vi "gm_mysql_write_gmvalues.vi"(7 "db connection":bool, 8 "error in (no error)":errorcluster, 10 "Output - Cluster gm":T3 {"GM TS-2[°C]" format="%.2g"; "GM TS-1 [°C]" format="%.2g"; "GM DS-1 [bar]" format="%.4g"; "GM DS-2 [bar]" format="%.4g"; "GA1 h2 [%]" format="%.2g"; "GA1 co2 [%]" format="%.2g"; "GA1 ch4 [%]" format="%.2g"}, 11 "log vars in":T1) -> (0 "error out":errorcluster, 2 "db connection":bool, 3 "log vars out":T1)   [LabVIEW 2011]
uses:
  Output - Cluster gas.ctl
  gas_values.ctl
  GM_host_db_log_vars.ctl
  <vilib>/addons/database/Connection.llb/Conn ObjectReference.ctl
  <vilib>/Utility/error.llb/DialogType.ctl
  <vilib>/addons/database/NI_Database_API.lvlib
panel:
  # "qualitätsmessung"
  # "quantitätsmessung"
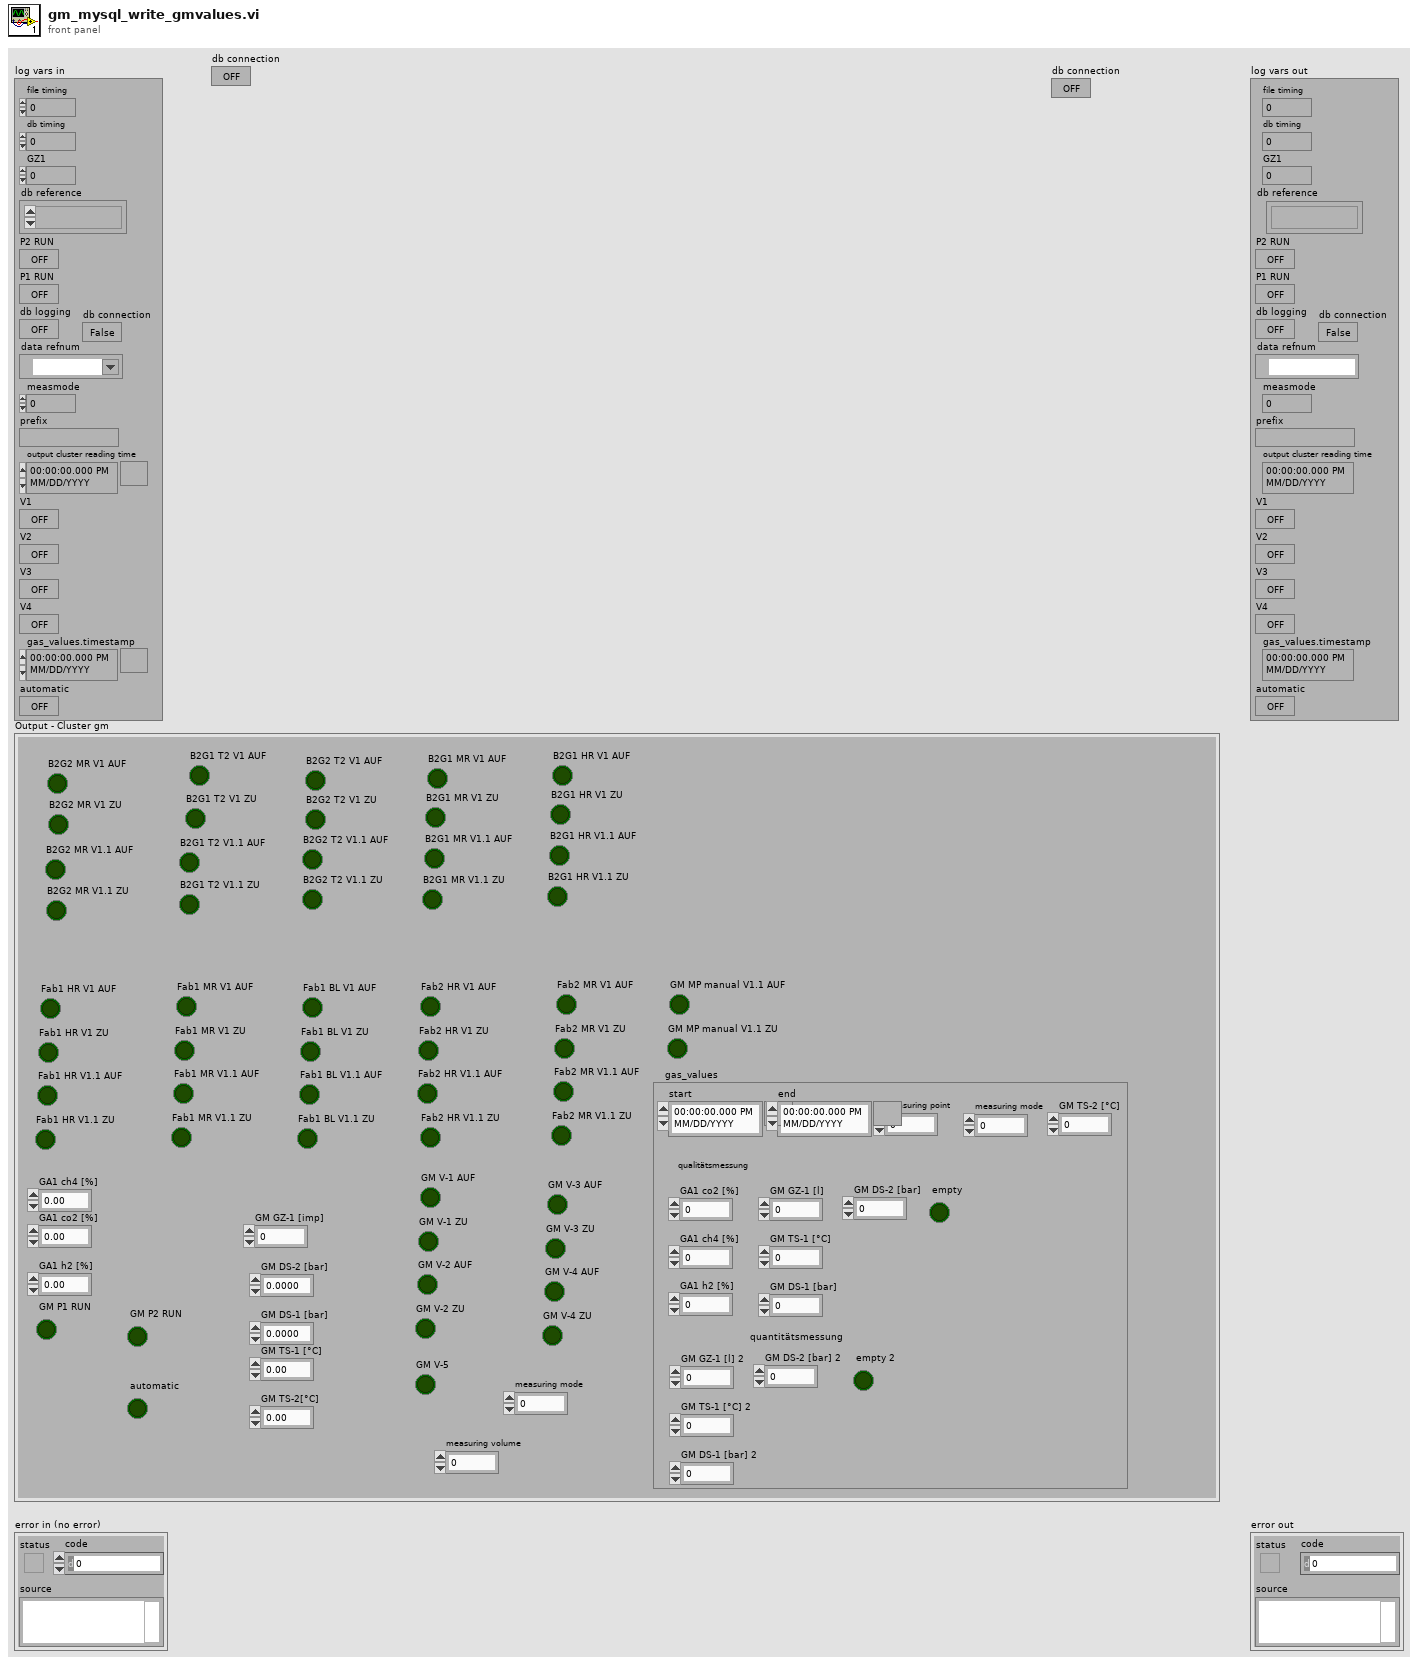
[diagram p1: front panel]
types:
  T1 = typedef "GM_host_db_log_vars.ctl" = cluster{"file timing":i64, "db timing":i64, "GZ1":u32, "db reference":T2, "P2 RUN":bool, "P1 RUN":bool, "db logging":bool, "data refnum":refnum<k21>, "measmode":u32, "prefix":string, "output cluster reading time":timestamp, "V1":bool, "V2":bool, "V3":bool, "V4":bool, "gas_values.timestamp":timestamp, "automatic":bool, "db connection":bool}
  T2 = typedef "NI_Database_API.lvlib/Conn ObjectReference.ctl" = refnum<k1>
  T3 = typedef "Output - Cluster gas.ctl" = cluster{"B2G2 MR V1.1 AUF":bool, "B2G2 MR V1.1 ZU":bool, "B2G2 MR V1 AUF":bool, "B2G2 MR V1 ZU":bool, "B2G1 T2 V1 AUF":bool, "B2G1 T2 V1 ZU":bool, "B2G1 T2 V1.1 AUF":bool, "B2G1 T2 V1.1 ZU":bool, "B2G2 T2 V1 AUF":bool, "B2G2 T2 V1 ZU":bool, "B2G2 T2 V1.1 ZU":bool, "B2G2 T2 V1.1 AUF":bool, "B2G1 MR V1 AUF":bool, "B2G1 MR V1 ZU":bool, "B2G1 MR V1.1 AUF":bool, "B2G1 MR V1.1 ZU":bool, "B2G1 HR V1 AUF":bool, "B2G1 HR V1 ZU":bool, "B2G1 HR V1.1 AUF":bool, "B2G1 HR V1.1 ZU":bool, "Fab1 HR V1 AUF":bool, "Fab1 HR V1 ZU":bool, "Fab1 HR V1.1 AUF":bool, "Fab1 HR V1.1 ZU":bool, "Fab1 MR V1 AUF":bool, "Fab1 MR V1 ZU":bool, "Fab1 MR V1.1 AUF":bool, "Fab1 MR V1.1 ZU":bool, "Fab1 BL V1 AUF":bool, "Fab1 BL V1 ZU":bool, "Fab1 BL V1.1 AUF":bool, "Fab1 BL V1.1 ZU":bool, "Fab2 HR V1 AUF":bool, "Fab2 HR V1 ZU":bool, "Fab2 HR V1.1 AUF":bool, "Fab2 HR V1.1 ZU":bool, "Fab2 MR V1 AUF":bool, "Fab2 MR V1 ZU":bool, "Fab2 MR V1.1 AUF":bool, "Fab2 MR V1.1 ZU":bool, "GA1 ch4 [%]":dbl, "GA1 co2 [%]":dbl, "GA1 h2 [%]":dbl, "GM P1 RUN":bool, "GM V-1 AUF":bool, "GM V-1 ZU":bool, "GM V-2 AUF":bool, "GM V-2 ZU":bool, "GM V-3 AUF":bool, "GM V-3 ZU":bool, "GM V-4 AUF":bool, "GM V-4 ZU":bool, "GM P2 RUN":bool, "GM GZ-1 [imp]":u32, "GM DS-2 [bar]":dbl, "GM DS-1 [bar]":dbl, "GM TS-1 [°C]":dbl, "GM TS-2[°C]":dbl, "gas_values":T4, "measuring mode":u8, "GM V-5":bool, "measuring volume":dbl, "automatic":bool, "GM MP manual V1.1 AUF":bool, "GM MP manual V1.1 ZU":bool}
  T4 = typedef "gas_values.ctl" = cluster{"start":timestamp, "GM DS-2 [bar]":dbl, "GA1 ch4 [%]":dbl, "GA1 co2 [%]":dbl, "GA1 h2 [%]":dbl, "GM DS-1 [bar]":dbl, "GM TS-1 [°C]":dbl, "GM TS-2 [°C]":dbl, "GM GZ-1 [l]":dbl, "measuring point":u8, "end":timestamp, "empty":bool, "GM GZ-1 [l] 2":dbl, "GM TS-1 [°C] 2":dbl, "GM DS-1 [bar] 2":dbl, "GM DS-2 [bar] 2":dbl, "empty 2":bool, "measuring mode":u8}
  T5 = typedef "DialogType.ctl" = u16
  T6 = cluster{"start":timestamp, "end":timestamp, "measuring point":u8, "measuring mode":u8, "GA1 co2 [%]":dbl, "GA1 ch4 [%]":dbl, "GA1 h2 [%]":dbl, "GM GZ-1 [l]":dbl, "GM DS-1 [bar]":dbl, "GM TS-1 [°C]":dbl, "GM DS-2 [bar]":dbl, i16, "GM TS-2 [°C]":dbl}
  T7 = cluster{"start":timestamp, "end":timestamp, "measuring point":u8, "measuring mode":u8, "GM GZ-1 [l] 2":dbl, "GM DS-1 [bar] 2":dbl, "GM TS-1 [°C] 2":dbl, "GM DS-2 [bar] 2":dbl, i16, "GM TS-2 [°C]":dbl}
  T8 = cluster{"start":timestamp, "end":timestamp, "measuring point":u8, "measuring mode":u8, "GA1 co2 [%]":dbl, "GA1 ch4 [%]":dbl, "GA1 h2 [%]":dbl, "GM GZ-1 [l]":dbl, "GM DS-1 [bar]":dbl, "GM TS-1 [°C]":dbl, "GM DS-2 [bar]":dbl, i16, "GM GZ-1 [l] 2":dbl, "GM DS-1 [bar] 2":dbl, "GM TS-1 [°C] 2":dbl, "GM DS-2 [bar] 2":dbl, i16, "GM TS-2 [°C]":dbl}
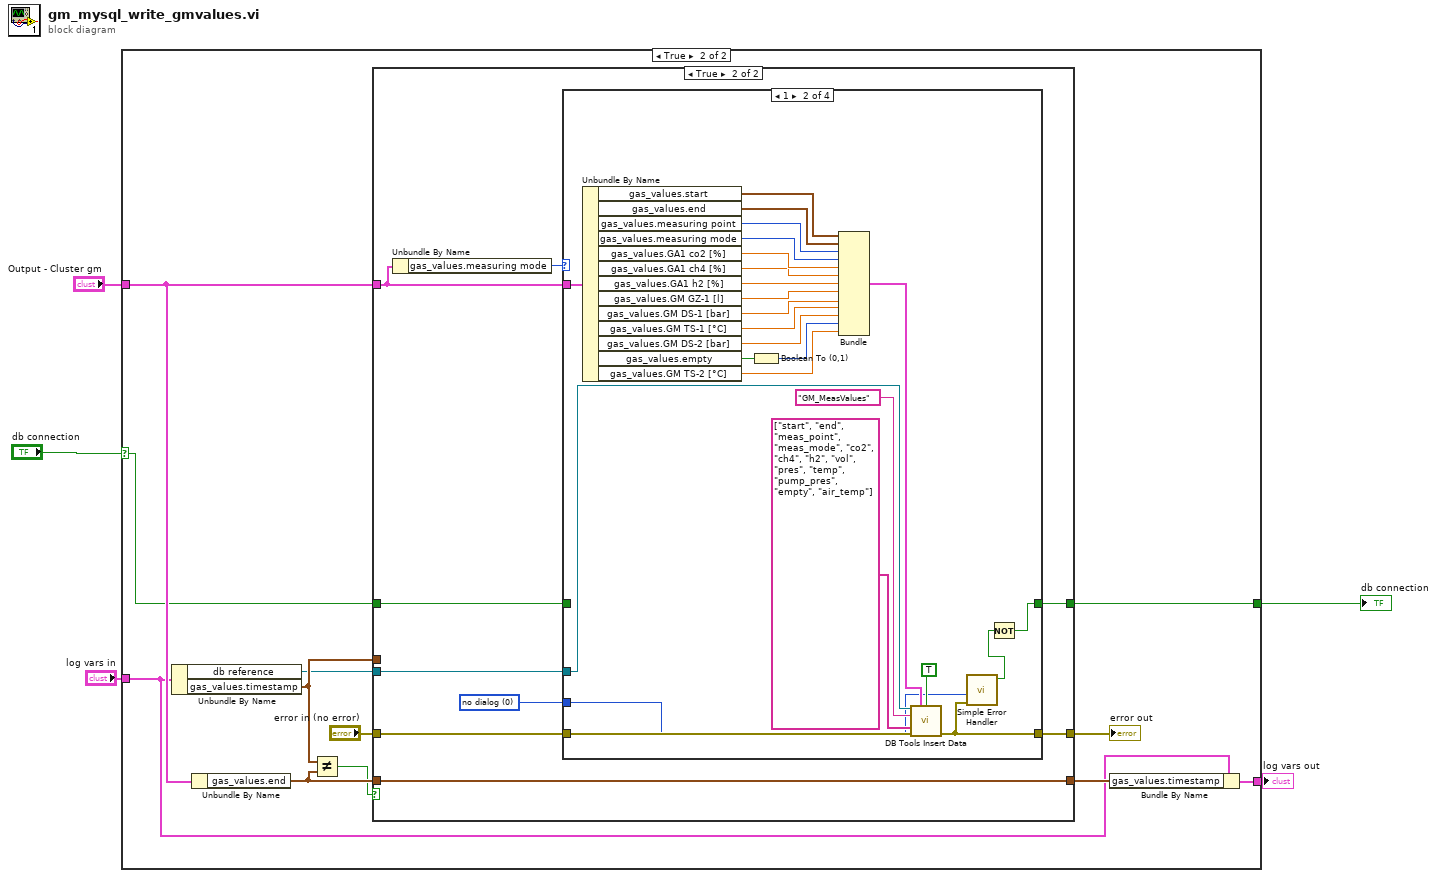
[diagram p0: block diagram]
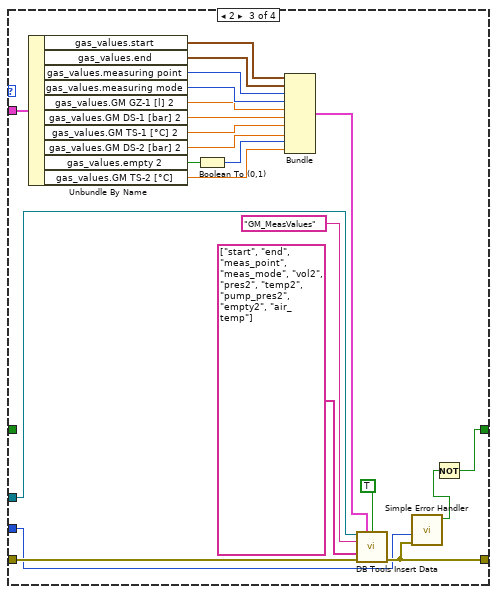
[diagram p5: hidden frame]
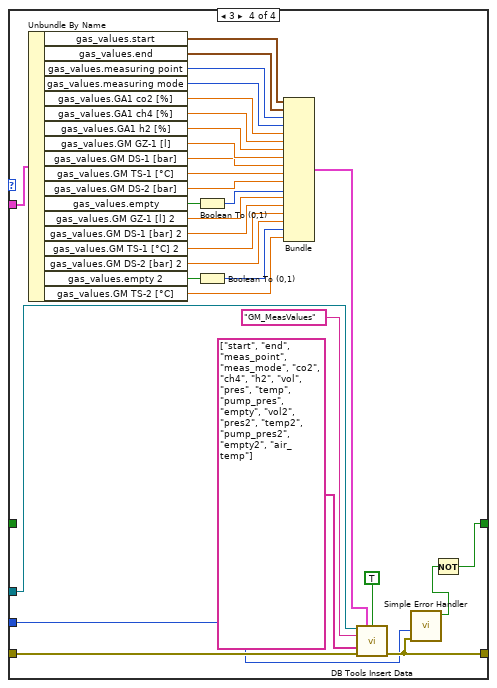
[diagram p6: hidden frame]
diagram:
  n1 = case shown="True" "db connection" {
    selector: "db connection" -> [w6 w8]
    tunnel: "Output - Cluster gm" -> [_ w14]
    tunnel: "log vars in" -> [w7 w13]
    tunnel: [w7 w10] -> w3
    tunnel: [w6 w9] -> w1
    frame False {
    }
    frame True {
      n2 = Unbundle By Name(w13) -> ("db reference"=w15:T2, "gas_values.timestamp"=w18:timestamp)
      n3 = Unbundle By Name(w14) -> ("gas_values.end"=w19:timestamp)
      n4 = Not Equal?(x=w18, y=w19) -> (x != y?=w16:bool)
      n5 = case shown="True" w16 {
        tunnel: "error in (no error)" -> [w21 w30]
        tunnel: [w21 w29] -> w12
        tunnel: w15 -> [_ w28]
        tunnel: [w22 w31] -> w17
        tunnel: w18 -> [w22 _]
        tunnel: w19 -> [_ w31]
        tunnel: w14 -> [_ w27]
        tunnel: [w20 w24] -> w9
        tunnel: w8 -> [w20 w23]
        frame False {
        }
        frame True {
          w25 = T5 0 items=["no dialog", "OK message", "continue or stop message", "OK message + warnings", "continue/stop + warnings"] ("type of dialog (OK msg:1)")
          n6 = Unbundle By Name(w27) -> ("gas_values.measuring mode"=w26:u8)
          n7 = case shown="1" w26 {
            tunnel: w30 -> [w33 w58 w80 w111]
            tunnel: [w33 w37 w61 w83] -> w29
            tunnel: w28 -> [_ w57 w79 w110]
            tunnel: w27 -> [_ w55 w77 w108]
            tunnel: w25 -> [_ w36 w60 w82]
            tunnel: [w32 w34 w59 w81] -> w24
            tunnel: w23 -> [w32 _ _ _]
            frame 0, Default {
            }
            frame 1 {
              n8 = Unbundle By Name(w55) -> ("gas_values.start"=w52:timestamp, "gas_values.end"=w51:timestamp, "gas_values.measuring point"=w50:u8, "gas_values.measuring mode"=w49:u8, "gas_values.GA1 co2 [%]"=w48:dbl, "gas_values.GA1 ch4 [%]"=w47:dbl, "gas_values.GA1 h2 [%]"=w46:dbl, "gas_values.GM GZ-1 [l]"=w45:dbl, "gas_values.GM DS-1 [bar]"=w44:dbl, "gas_values.GM TS-1 [°C]"=w43:dbl, "gas_values.GM DS-2 [bar]"=w42:dbl, "gas_values.empty"=w41:bool, "gas_values.GM TS-2 [°C]"=w39:dbl)
              n9 = Boolean To (0,1)(Boolean=w41) -> (0, 1=w40:i16)
              n10 = Bundle("start"=w52, "end"=w51, "measuring point"=w50, "measuring mode"=w49, "GA1 co2 [%]"=w48, "GA1 ch4 [%]"=w47, "GA1 h2 [%]"=w46, "GM GZ-1 [l]"=w45, "GM DS-1 [bar]"=w44, "GM TS-1 [°C]"=w43, "GM DS-2 [bar]"=w42, w40, "GM TS-2 [°C]"=w39) -> (w56:T6)  [unwired: 1 in]
              n11 = call <vilib>:"DB Tools Insert Data.vi"("connection reference"=w57, "data"=w56, "insert ignore? (F)"=TRUE, "table"="GM_MeasValues", "columns"=string[] ["start", "end", "meas_point", "meas_mode", "co2", "ch4", "h2", "vol", "pres", "temp", "pump_pres", "empty", "air_temp"], "error in (no error)"=w58) -> ("error out"=w37:errorcluster)  [unwired: 8 in, 1 out]
              n12 = call <vilib>:"Simple Error Handler.vi"("type of dialog (OK msg:1)"=w36, "error in (no error)"=w37) -> ("error?"=w35:bool)  [unwired: 3 in, 4 out]
              n13 = Not(x=w35) -> (.not. x?=w34:bool)
            }
            frame 2 {
              n14 = Unbundle By Name(w77) -> ("gas_values.start"=w74:timestamp, "gas_values.end"=w73:timestamp, "gas_values.measuring point"=w72:u8, "gas_values.measuring mode"=w71:u8, "gas_values.GM GZ-1 [l] 2"=w70:dbl, "gas_values.GM DS-1 [bar] 2"=w69:dbl, "gas_values.GM TS-1 [°C] 2"=w68:dbl, "gas_values.GM DS-2 [bar] 2"=w67:dbl, "gas_values.empty 2"=w66:bool, "gas_values.GM TS-2 [°C]"=w65:dbl)
              n15 = Boolean To (0,1)(Boolean=w66) -> (0, 1=w64:i16)
              n16 = Bundle("start"=w74, "end"=w73, "measuring point"=w72, "measuring mode"=w71, "GM GZ-1 [l] 2"=w70, "GM DS-1 [bar] 2"=w69, "GM TS-1 [°C] 2"=w68, "GM DS-2 [bar] 2"=w67, w64, "GM TS-2 [°C]"=w65) -> (w78:T7)  [unwired: 1 in]
              n17 = call <vilib>:"DB Tools Insert Data.vi"("connection reference"=w79, "data"=w78, "insert ignore? (F)"=TRUE, "table"="GM_MeasValues", "columns"=string[] ["start", "end", "meas_point", "meas_mode", "vol2", "pres2", "temp2", "pump_pres2", "empty2", "air_temp"], "error in (no error)"=w80) -> ("error out"=w61:errorcluster)  [unwired: 8 in, 1 out]
              n18 = call <vilib>:"Simple Error Handler.vi"("type of dialog (OK msg:1)"=w60, "error in (no error)"=w61) -> ("error?"=w62:bool)  [unwired: 3 in, 4 out]
              n19 = Not(x=w62) -> (.not. x?=w59:bool)
            }
            frame 3 {
              n20 = Unbundle By Name(w108) -> ("gas_values.start"=w105:timestamp, "gas_values.end"=w104:timestamp, "gas_values.measuring point"=w103:u8, "gas_values.measuring mode"=w102:u8, "gas_values.GA1 co2 [%]"=w101:dbl, "gas_values.GA1 ch4 [%]"=w100:dbl, "gas_values.GA1 h2 [%]"=w99:dbl, "gas_values.GM GZ-1 [l]"=w98:dbl, "gas_values.GM DS-1 [bar]"=w97:dbl, "gas_values.GM TS-1 [°C]"=w96:dbl, "gas_values.GM DS-2 [bar]"=w95:dbl, "gas_values.empty"=w94:bool, "gas_values.GM GZ-1 [l] 2"=w93:dbl, "gas_values.GM DS-1 [bar] 2"=w92:dbl, "gas_values.GM TS-1 [°C] 2"=w91:dbl, "gas_values.GM DS-2 [bar] 2"=w90:dbl, "gas_values.empty 2"=w89:bool, "gas_values.GM TS-2 [°C]"=w88:dbl)
              n21 = Boolean To (0,1)(Boolean=w94) -> (0, 1=w86:i16)
              n22 = Boolean To (0,1)(Boolean=w89) -> (0, 1=w87:i16)
              n23 = Bundle("start"=w105, "end"=w104, "measuring point"=w103, "measuring mode"=w102, "GA1 co2 [%]"=w101, "GA1 ch4 [%]"=w100, "GA1 h2 [%]"=w99, "GM GZ-1 [l]"=w98, "GM DS-1 [bar]"=w97, "GM TS-1 [°C]"=w96, "GM DS-2 [bar]"=w95, w86, "GM GZ-1 [l] 2"=w93, "GM DS-1 [bar] 2"=w92, "GM TS-1 [°C] 2"=w91, "GM DS-2 [bar] 2"=w90, w87, "GM TS-2 [°C]"=w88) -> (w109:T8)  [unwired: 1 in]
              n24 = call <vilib>:"DB Tools Insert Data.vi"("connection reference"=w110, "data"=w109, "insert ignore? (F)"=TRUE, "table"="GM_MeasValues", "columns"=string[] ["start", "end", "meas_point", "meas_mode", "co2", "ch4", "h2", "vol", "pres", "temp", "pump_pres", "empty", "vol2", "pres2", "temp2", "pump_pres2", "empty2", "air_temp"], "error in (no error)"=w111) -> ("error out"=w83:errorcluster)  [unwired: 8 in, 1 out]
              n25 = call <vilib>:"Simple Error Handler.vi"("type of dialog (OK msg:1)"=w82, "error in (no error)"=w83) -> ("error?"=w84:bool)  [unwired: 3 in, 4 out]
              n26 = Not(x=w84) -> (.not. x?=w81:bool)
            }
          }
        }
      }
      "error out" <- w12
      n27 = Bundle By Name(cluster=w13, "gas_values.timestamp"=w17) -> (w10:T1)
    }
  }
  "log vars out" <- w3
  "db connection" <- w1
